vi "GetBufferTimestampResolution.vi"(7 "SMU":T1, 8 "Error In":errorcluster, 10 "Buffer":u8=1 min=1 max=2 step=1, 11 "Kiethley 2602 In":refnum<visa-resource-name>) -> (0 "Error Out":errorcluster, 2 "Resolution (sec)":dbl, 3 "Keithley 2602 Out":refnum<visa-resource-name>)   [LabVIEW 2012, in "Keithley-2602.lvlib"]
uses:
  Keithley-2602.lvlib
  Controls/SMU.ctl
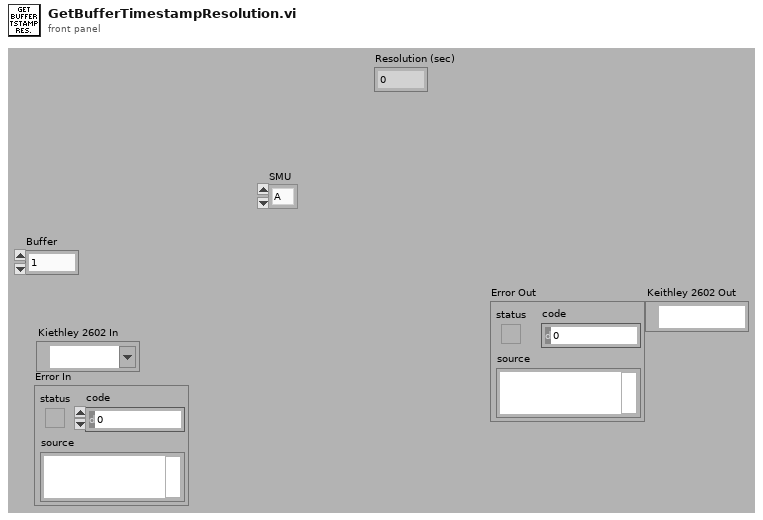
[diagram p1: front panel]
types:
  T1 = typedef "Keithley-2602.lvlib/SMU.ctl" = enum16{"A", "B"}
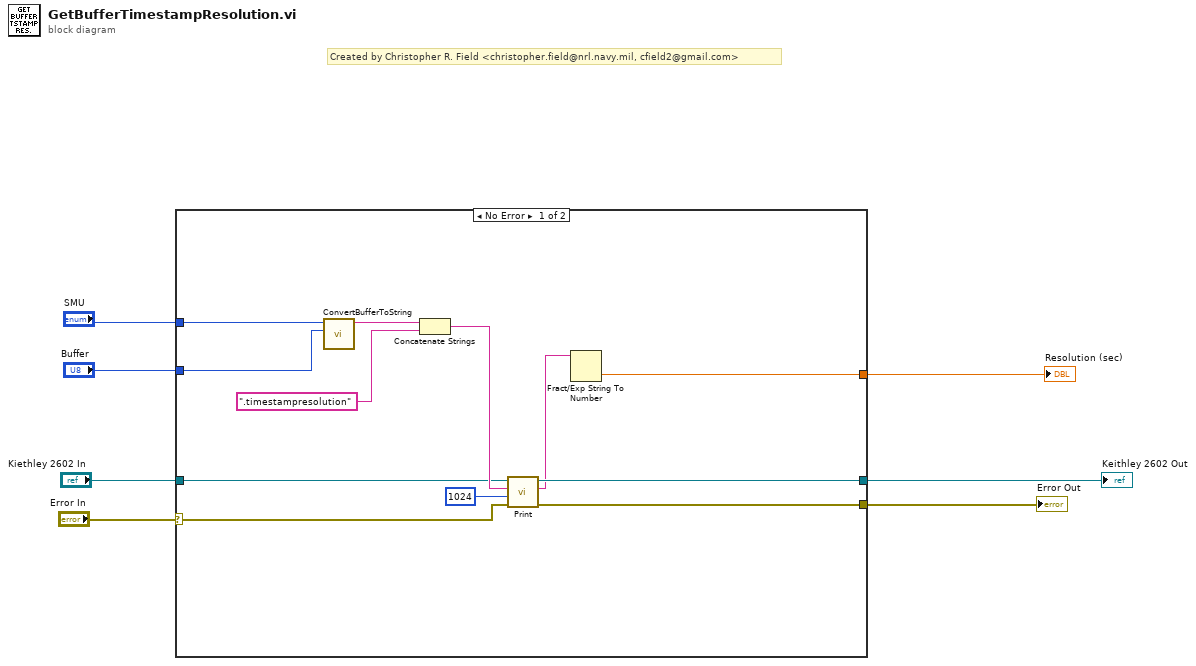
[diagram p0: block diagram]
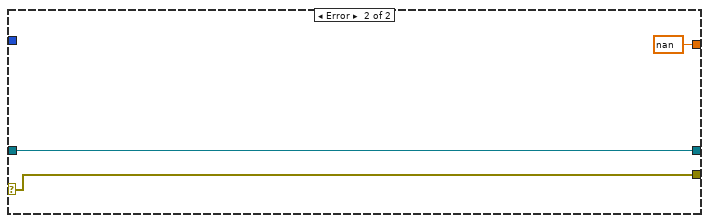
[diagram p2: hidden frame]
diagram:
  # "Created by Christopher R. Field <christopher.field@nrl.navy.mil, cfield2@gmail.com>"
  n1 = case shown="No Error" "Error In" {
    selector: "Error In" -> [w8 w22]
    tunnel: "Kiethley 2602 In" -> [w17 w21]
    tunnel: [w16 w22] -> w6
    tunnel: [w15 w21] -> w5
    tunnel: "Buffer" -> [w13 _]
    tunnel: [w10 nan] -> w3
    tunnel: "SMU" -> [w9 _]
    frame No Error {
      n2 = call "ConvertBufferToString.vi"("Buffer"=w13, "SMU"=w9) -> ("Buffer"=w12:string)  [unwired: 9 in]
      n3 = Concatenate Strings(w12, ".timestampresolution" ("string")) -> (w19:string)
      n4 = call "Print.vi"("Error In"=w8, "Byte Count"=u32 1024, "Attribute"=w19, "Kiethley 2602 In"=w17) -> ("Error Out"=w16:errorcluster, "Output"=w14:string, "Keithley 2602 Out"=w15:refnum<visa-resource-name>)  [unwired: 5 in]
      n5 = Fract/Exp String To Number(string=w14) -> (number=w10:dbl)  [unwired: 3 in, 1 out]
    }
    frame Error {
    }
  }
  "Error Out" <- w6
  "Keithley 2602 Out" <- w5
  "Resolution (sec)" <- w3
